vi "SMU_Meas_Voltage_Simple.vi"(8 "error in (no error)":errorcluster, 10 "Pins":string[](array[string])=["VDD"], 11 "Semiconductor Module Context":T1) -> (0 "error out":errorcluster, 3 "HV_Measurement":dbl)   [LabVIEW 2013]
uses:
  <vilib>/NI_TestStand_SemiconductorModule/NI_TestStand_Semiconductor_Module.lvlibp/PinMap/General/SemiconductorModuleContext.ctl
  <vilib>/NI_TestStand_SemiconductorModule/NI_TestStand_Semiconductor_Module.lvlibp/PinMap/DC Power/PinsToNIDCPowerSessions.vi
  <vilib>/NI_TestStand_SemiconductorModule/NI_TestStand_Semiconductor_Module.lvlibp
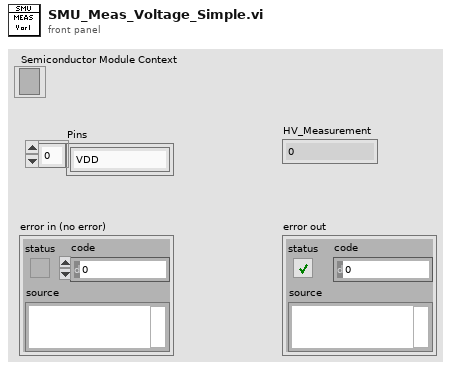
[diagram p1: front panel]
types:
  T1 = typedef "NI_TestStand_Semiconductor_Module.lvlibp/SemiconductorModuleContext.ctl" = refnum<k7>
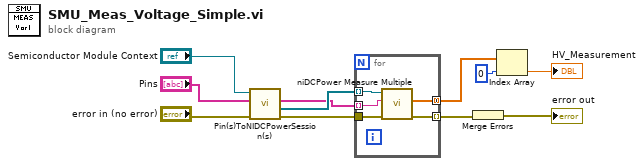
[diagram p0: block diagram]
diagram:
  n1 = call-poly <vilib>:"Pin(s)ToNIDCPowerSession(s).vi"("error in (no error)"="error in (no error)", "Pins"="Pins", "Semiconductor Module Context"="Semiconductor Module Context") -> ("error out"=w5:errorcluster, "Instrument Sessions"=w7:refnum<k15>[], "Channel Lists"=w6:string[])  [unwired: 4 in, 2 out]
  n2 = for {
    tunnel: w7 -> [w16] mode=indexing
    tunnel: w6 -> [w15] mode=indexing
    tunnel: w5 -> [w14]
    tunnel: [w13] -> w4 mode=indexing
    tunnel: [w12] -> w3 mode=concatenating
    n3 = call <instrlib>:"niDCPower Measure Multiple.vi"("error in (no error)"=w14, "channel name"=w15, "instrument handle"=w16) -> ("error out"=w13:errorcluster, "voltage measurements"=w12:dbl[])  [unwired: 5 in, 2 out]
  }
  n4 = Merge Errors(w4) -> (→"error out":errorcluster)
  n5 = Index Array(array=w3, index=0) -> (element=→"HV_Measurement":dbl)
